vi "GEN_Speed-coded_overlay_PIC.vi"(6 "Speed array in":dbl[](array[numeric]), 7 "Image size":cluster{"x":i32, "y":i32}={"x"=480, "y"=480}, 8 "Error In":errorcluster, 9 "Samples full merge, every N":i32=10000, 10 "Multiline grouping, samples":i32=100, 11 "Full track array":T1(array[cluster])) -> (0 "Error Out":errorcluster, 3 "Speed-coded overlay pixmap":u32[][](array[numeric]) format="%x")   [LabVIEW 2018, in "Tracker.lvlib"]
uses:
  Tracker.lvlib
  Controls/CTL_Color_ramp.ctl
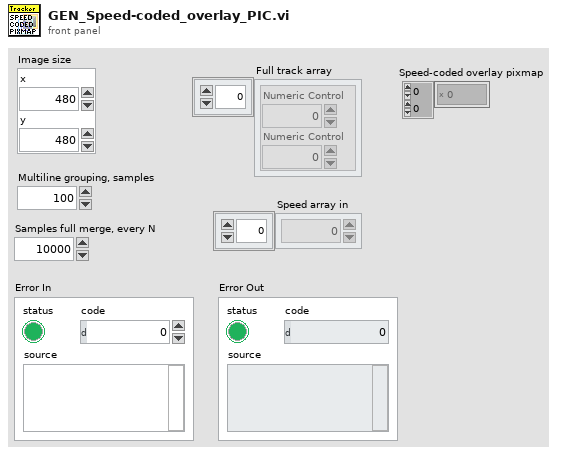
[diagram p1: front panel]
types:
  T1 = cluster{"Numeric Control":dbl, "Numeric Control":dbl}[]
  T2 = typedef "Tracker.lvlib/CTL_Color_ramp.ctl" = u32[]
  T3 = cluster{"Left":i32, "Top":i32, "Right":i32, "Bottom":i32}
  T4 = cluster{"Width":i16, "Style":enum32{"Solid", "Dash", "Dot", "DashDot", "DashDotDot"}}
  T5 = cluster{"Numeric Control":dbl, "Numeric Control":dbl}
  T6 = cluster{"Width":u16, "Style":enum32{"Solid", "Dash", "Dot", "DashDot", "DashDotDot"}}
  T7 = typedef "imagedata.ctl" = cluster{"image type":i32, "image depth":i32, "image":u8[], "mask":u8[], "colors":u32[], "Rectangle":cluster{"left":i16, "top":i16, "right":i16, "bottom":i16}}
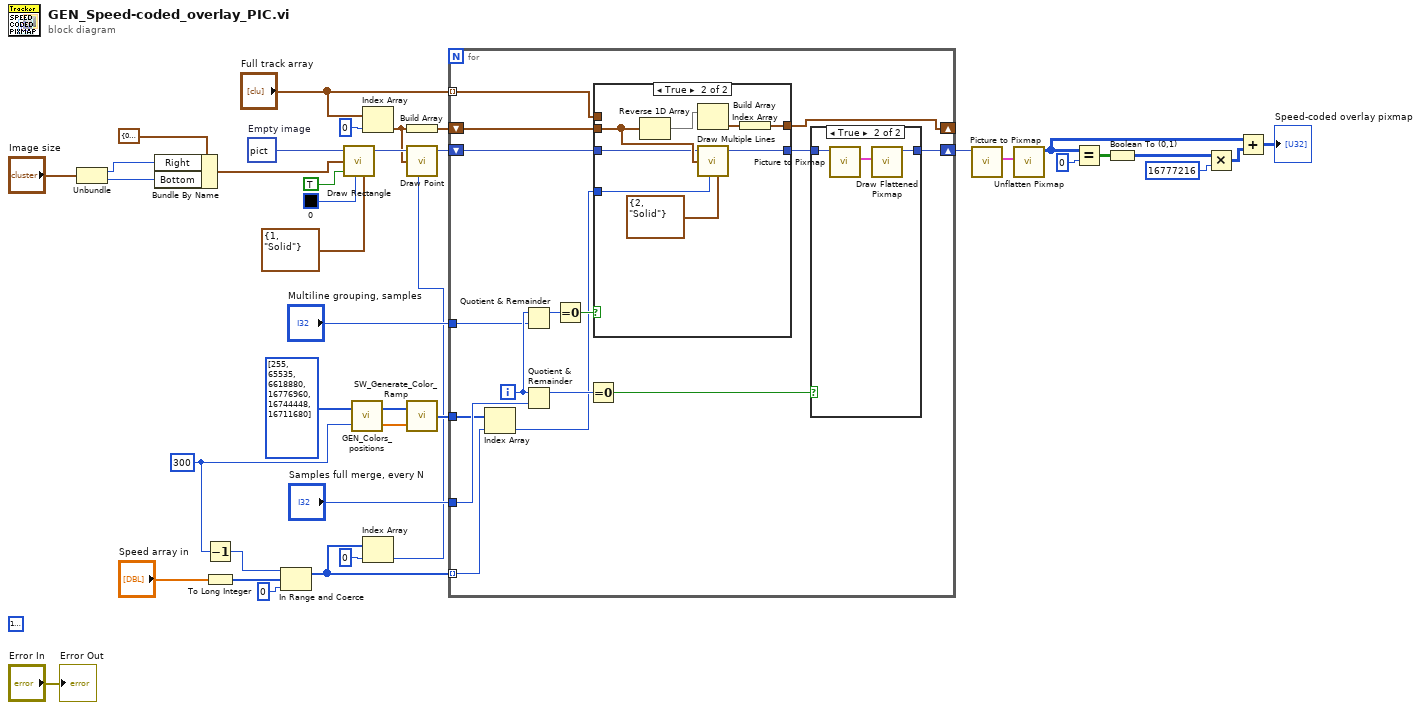
[diagram p0: block diagram]
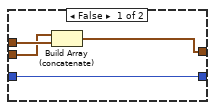
[diagram p2: hidden frame]
diagram:
  w4 = 300
  (unwired) u32 16777216
  w25 = picture data[5B]  # Empty image
  n1 = Unbundle("Image size") -> ("x"=w37:i32, "y"=w38:i32)
  n2 = Bundle By Name(cluster=T3 {"Left"=0, "Top"=0, "Right"=0, "Bottom"=0} ("Rectangle"), "Right"=w37, "Bottom"=w38) -> (w39:T3)
  n3 = Decrement(x=w4) -> (x-1=w5:i32)
  n4 = To Long Integer(number="Speed array in") -> (32bit integer=w7:i32[])
  n5 = In Range and Coerce(upper limit=w5, x=w7, lower limit=0) -> (coerced(x)=w1:i32[])  [unwired: 1 out]
  n6 = call <vilib>:"Draw Rectangle.vi"("picture"=w25, "rect"=w39, "fill?(F)"=TRUE, "color(black)"=u32 0, "pen"=T4 {"Width"=1, "Style"=enum."Solid"}) -> ("new picture"=w34:picture)  [unwired: 4 in]
  n7 = call "GEN_Colors_positions.vi"("Highest color position"=w4, "Initial colors ramp array in"=T2 [255, 65535, 6618880, 16776960, 16744448, 16711680] ("Initial colors ramp array")) -> ("Colors positions"=w22:dbl[], "Initial colors ramp array out"=w23:T2)
  n8 = Index Array(array="Full track array", index=0) -> (element=w29:T5)
  n9 = Index Array(array=w1, index=0) -> (element=w2:i32)
  n10 = Build Array(w29) -> (w30:T1)
  n11 = call <vilib>:"Draw Point.vi"("picture"=w34, "point(x,y)"=w29, "color(black)"=w2) -> ("new picture"=w28:picture)  [unwired: 6 in]
  n12 = call "SW_Generate_Color_Ramp.vi"("Colors rel. pos."=w22, "Colors array"=w23) -> ("Colors array"=w19:u32[])
  n13 = for {
    shift-right: [w52] -> w31
    shift-left: w28 -> [w51]
    tunnel: "Full track array" -> [w46] mode=indexing
    tunnel: w19 -> [w42]
    tunnel: "Samples full merge, every N" -> [w53]
    tunnel: "Multiline grouping, samples" -> [w48]
    shift-right: [w44] -> _
    shift-left: w30 -> [w45]
    tunnel: w1 -> [w41] mode=indexing
    i -> [w49]
    n14 = Index Array(array=w42, index=w41) -> (element=w40:u32)
    n15 = Quotient & Remainder(x=w49, y=w48) -> (x-y*floor(x/y)=w50:i32)  [unwired: 1 out]
    n16 = Quotient & Remainder(x=w49, y=w53) -> (x-y*floor(x/y)=w54:i32)  [unwired: 1 out]
    n17 = Equal To 0?(x=w50) -> (x = 0?=w43:bool)
    n18 = Equal To 0?(x=w54) -> (x = 0?=w55:bool)
    n19 = case shown="True" w43 {
      tunnel: w51 -> [w59 w62]
      tunnel: [w59 w61] -> w47
      tunnel: w46 -> [w58 _]
      tunnel: w45 -> [w57 w63]
      tunnel: [w56 w60] -> w44
      tunnel: w40 -> [_ w64]
      frame False {
        n20 = Build Array (concatenate)(w57, w58) -> (w56:T1)
      }
      frame True {
        n21 = Reverse 1D Array(array=w63) -> (reversed array=w67:T1)
        n22 = Index Array(array=w67) -> (element=w66:T5)  [unwired: 1 in]
        n23 = call <vilib>:"Draw Multiple Lines.vi"("picture"=w62, "line endpoints"=w63, "color(black)"=w64, "pen"=T6 {"Width"=2, "Style"=enum."Solid"}) -> ("new picture"=w61:picture)  [unwired: 5 in]
        n24 = Build Array(w66) -> (w60:T1)
      }
    }
    n25 = case shown="True" w55 {
      tunnel: [w68 w70] -> w52
      tunnel: w47 -> [w68 w69]
      frame False {
      }
      frame True {
        n26 = call <vilib>:"Picture to Pixmap.vi"("picture"=w69) -> ("image data"=w71:T7)  [unwired: 9 in, 1 out]
        n27 = call <vilib>:"Draw Flattened Pixmap.vi"("image data"=w71) -> ("new picture"=w70:picture)  [unwired: 8 in]
      }
    }
  }
  n28 = call <vilib>:"Picture to Pixmap.vi"("picture"=w31) -> ("image data"=w18:T7)  [unwired: 9 in, 1 out]
  n29 = call <vilib>:"Unflatten Pixmap.vi"("image data"=w18) -> ("24-bit pixmap"=w10:u32[][])  [unwired: 4 in, 6 out]
  n30 = Equal?(x=w10, y=0) -> (x = y?=w14:bool[][])
  n31 = Boolean To (0,1)(Boolean=w14) -> (0, 1=w13:i16[][])
  n32 = Multiply(x=w13, y=16777216) -> (x*y=w11:i32[][])
  n33 = Add(x=w10, y=w11) -> (x+y=→"Speed-coded overlay pixmap":u32[][])
  "Error Out" <- "Error In"
